vi "MessageName.vi"() -> (2 "MessageName":string)   [LabVIEW 2020, in "Discovery.lvlib"]
uses:
  Discovery.lvlib
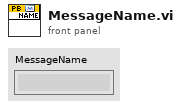
[diagram p1: front panel]
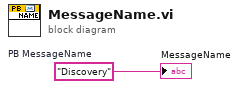
[diagram p0: block diagram]
diagram:
  w1 = "Discovery"  # PB MessageName
  "MessageName" <- w1
